vi "GF_ConfigPCIe6535.vi"() -> (0 "PCIE-ShotQSwitch":refnum<k21>="USB-MagAndTrigFire", 3 "PCIE-FastFire":refnum<k21>="USB-MagAndTrigFire")   [LabVIEW 2016]
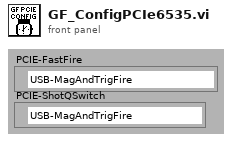
[diagram p1: front panel]
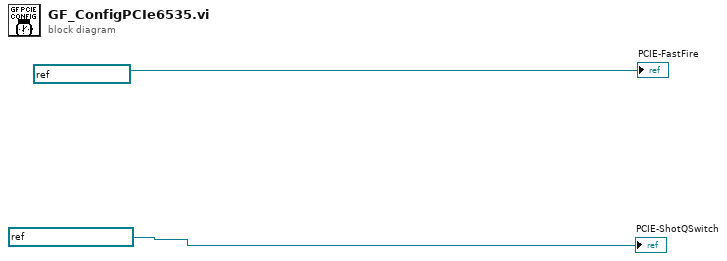
[diagram p0: block diagram]
diagram:
  "PCIE-FastFire" <- refnum<k21> "PCIE-FastFire" ("DAQmx Task Name")
  "PCIE-ShotQSwitch" <- refnum<k21> "PCIE-ShotQSwitch" ("DAQmx Task Name 2")
